vi "FPGA.vi"() -> ()   [LabVIEW 2014]
uses:
  <vilib>/rvi/Emulation/niFpgaGetClockAttributes.vi
  <vilib>/rvi/Emulation/niFpgaSctlEmulationGetInTimedLoop.vi
  <vilib>/rvi/Emulation/niFpgaEmulationReportErrorSimple.vi
  <vilib>/rvi/eio/common/nirviEmuTemplateMethod_errors.vi
  <vilib>/rvi/Emulation/niFpgaCriticalErrorInLSC.vi
  <vilib>/eio/EIONode/EIONode.xnode
panel:
  out "Chassis Temperature":sgl format="%.6f"
  in  "Desired Temperature Units":i16(ring) items=["Celsius", "Fahrenheit", "Kelvin", "Rankine"]
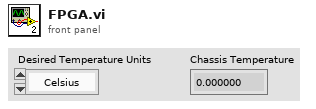
[diagram p1: front panel]
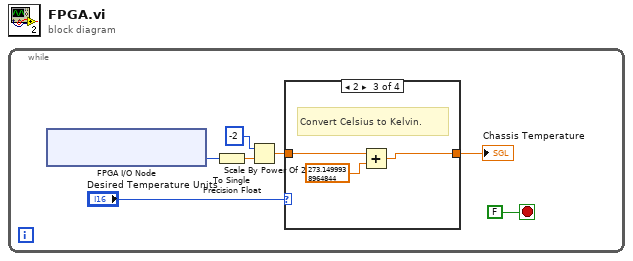
[diagram p0: block diagram]
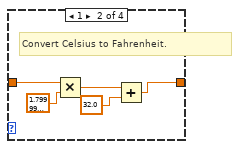
[diagram p3: hidden frame]
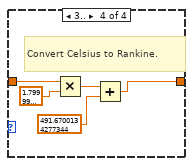
[diagram p4: hidden frame]
diagram:
  n1 = while {
    stop <- FALSE stop-if-true
    n2 = xnode "FPGA I/O Node"() -> ("Chassis Temperature"=w2:i16)  [unwired: 1 in, 1 out]
    n3 = To Single Precision Float(number=w2) -> (single precision float=w4:sgl)
    n4 = Scale By Power Of 2(n=i16 -2, x=w4) -> (x*2^n=w1:sgl)
    n5 = case shown="2" "Desired Temperature Units" {
      tunnel: w1 -> [w8 w13 w15 w18]
      tunnel: [w8 w9 w14 w17] -> w5
      frame ..0 {
        # "Leave value as Celsius."
      }
      frame 1 {
        # "Convert Celsius to Fahrenheit."
        n6 = Multiply(x=w13, y=sgl 1.8) -> (x*y=w11:sgl)
        n7 = Add(x=w11, y=sgl 32.0) -> (x+y=w9:sgl)
      }
      frame 2 {
        # "Convert Celsius to Kelvin."
        n8 = Add(x=w15, y=sgl 273.15) -> (x+y=w14:sgl)
      }
      frame 3.. {
        # "Convert Celsius to Rankine."
        n9 = Multiply(x=w18, y=sgl 1.8) -> (x*y=w20:sgl)
        n10 = Add(x=w20, y=sgl 491.67) -> (x+y=w17:sgl)
      }
    }
    "Chassis Temperature" <- w5
  }
